vi "Rapid Target Adjustment.vi"(0 "Focus and Tracking":T4, 1 "Calibration":T2, 2 "Target":T1, 3 "System of Reference Interface":T3, 4 "Tip":T5, 5 "Error In":errorcluster, 6 "Step [um]":dbl=4.0, 7 "Contrast AVG frames number [unused]":i32=3, 10 "Max Distance [um]":dbl=100.0, 11 "Active":refnum<vi>, 12 "Start Coordinates [pix]":refnum<vi>, 13 "Abort":refnum<vi>) -> (14 "Fail":bool, 15 "Scope Error":bool, 17 "Aborted":bool, 18 "Optical Coordinates [um]":cluster{"X":dbl, "Y":dbl, "Z":dbl}, 19 "Error Out":errorcluster)   [LabVIEW 2012, in "Targeting Unit.lvlib"]
uses:
  Targeting Unit.lvlib
  <vilib>/Analysis/Matrix/Datatypes/RealMatrix.ctl
  <vilib>/Analysis/Matrix/NI_Matrix.lvlib
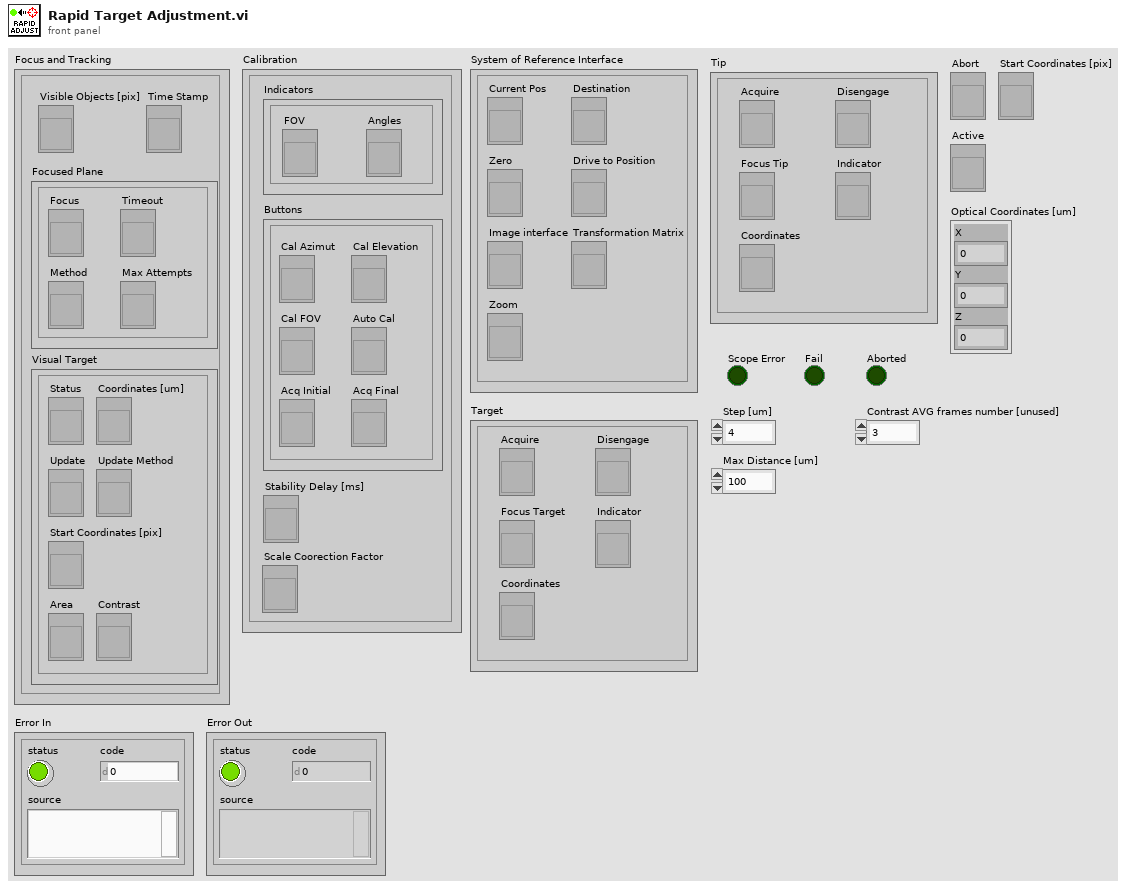
[diagram p1: front panel]
types:
  T1 = cluster{"Coordinates":refnum<vi>, "Acquire":refnum<vi>, "Disengage":refnum<vi>, "Indicator":refnum<vi>, "Focus Target":refnum<vi>}
  T2 = cluster{"Indicators":cluster{"FOV":refnum<vi>, "Angles":refnum<vi>}, "Buttons":cluster{"Cal FOV":refnum<vi>, "Cal Azimut":refnum<vi>, "Cal Elevation":refnum<vi>, "Auto Cal":refnum<vi>, "Acq Initial":refnum<vi>, "Acq Final":refnum<vi>}, "Stability Delay [ms]":refnum<vi>, "Scale Coorection Factor":refnum<vi>}
  T3 = cluster{"Current Pos":refnum<vi>, "Image interface":refnum<vi>, "Transformation Matrix":refnum<vi>, "Zero":refnum<vi>, "Destination":refnum<vi>, "Drive to Position":refnum<vi>, "Zoom":refnum<vi>}
  T4 = cluster{"Focused Plane":cluster{"Focus":refnum<vi>, "Timeout":refnum<vi>, "Max Attempts":refnum<vi>, "Method":refnum<vi>}, "Time Stamp":refnum<vi>, "Visual Target":cluster{"Coordinates [um]":refnum<vi>, "Status":refnum<vi>, "Update":refnum<vi>, "Update Method":refnum<vi>, "Start Coordinates [pix]":refnum<vi>, "Area":refnum<vi>, "Contrast":refnum<vi>}, "Visible Objects [pix]":refnum<vi>}
  T5 = cluster{"Coordinates":refnum<vi>, "Acquire":refnum<vi>, "Disengage":refnum<vi>, "Indicator":refnum<vi>, "Focus Tip":refnum<vi>}
  T6 = cluster{"X [um]":dbl, "Y [um]":dbl, "Z [um]":dbl}
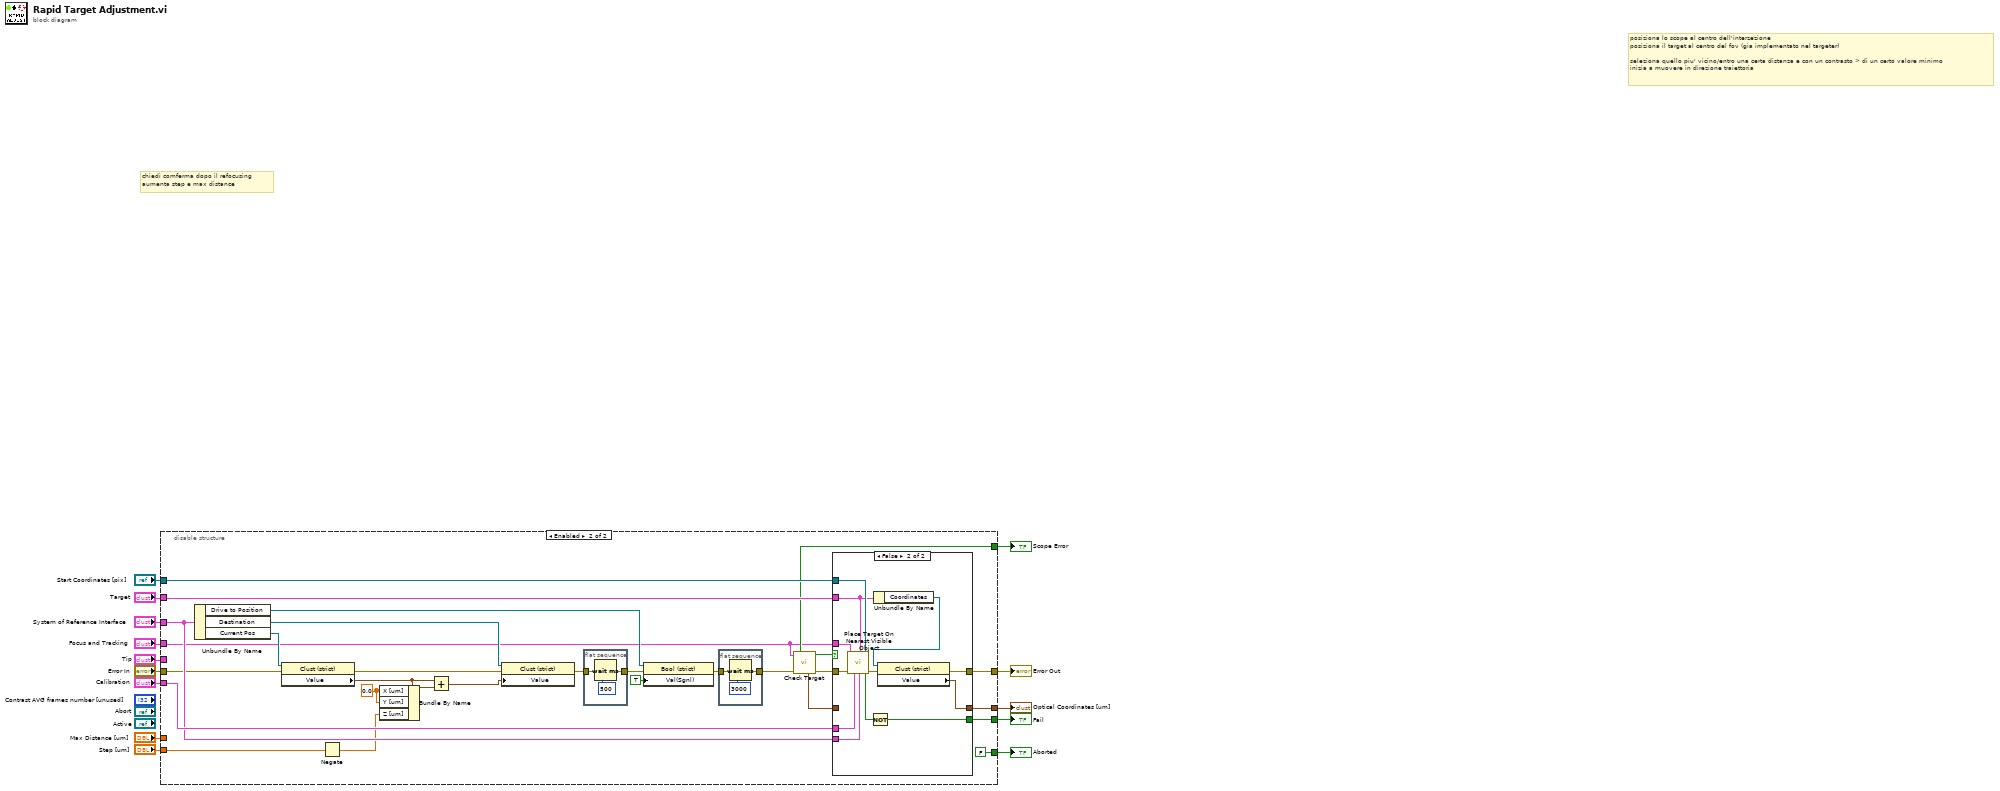
[diagram p0: block diagram]
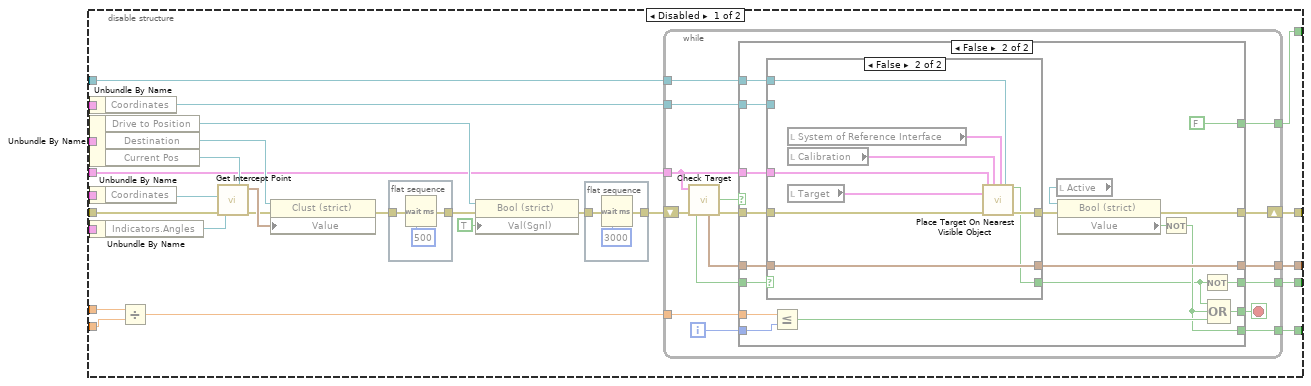
[diagram p2: hidden frame]
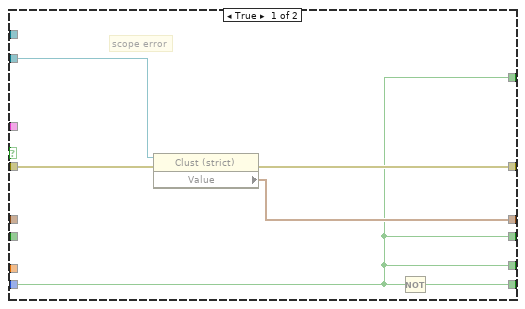
[diagram p3: hidden frame]
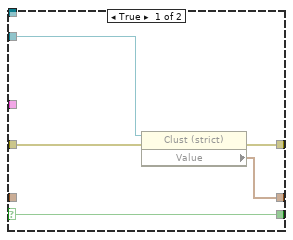
[diagram p4: hidden frame]
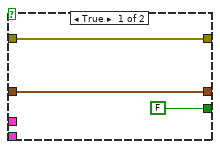
[diagram p5: hidden frame]
diagram:
  # "posiziona lo scope al centro dell'interzezione\nposiziona il target al centro del fov (gia implementato nel targeter)\n\nseleziona quello piu' vicino/entro una certa distanza e con un contrasto > di un certo valore minimo\ninizia a muovere in direzione traiettoria"
  # "chiedi comferma dopo il refocusing\naumenta step e max distance"
  n1 = disable-structure shown="Enabled" {
    disable-tunnel: "Step [um]" -> [w42 w112]
    disable-tunnel: "Max Distance [um]" -> [w41 _]
    disable-tunnel: "System of Reference Interface" -> [w40 w119]
    disable-tunnel: "Calibration" -> [w39 w120]
    disable-tunnel: "Tip" -> [w37 _]
    disable-tunnel: "Focus and Tracking" -> [w25 w102]
    disable-tunnel: [w24 FALSE ("Aborted")] -> w8
    disable-tunnel: [w23 w106] -> w7
    disable-tunnel: [w22 w127] -> w6
    disable-tunnel: "Target" -> [w21 w129]
    disable-tunnel: [w20 w105] -> w4
    disable-tunnel: [w19 w128] -> w3
    disable-tunnel: "Start Coordinates [pix]" -> [w15 w130]
    disable-tunnel: "Error In" -> [w26 w117]
    frame Disabled {
      n2 = Unbundle By Name(w21) -> ("Coordinates"=w18:refnum<vi>)
      n3 = Unbundle By Name(w40) -> ("Drive to Position"=w29:refnum<vi>, "Destination"=w30:refnum<vi>, "Current Pos"=w31:refnum<vi>)
      n4 = Unbundle By Name(w37) -> ("Coordinates"=w17:refnum<vi>)
      n5 = Unbundle By Name(w39) -> ("Indicators.Angles"=w27:refnum<vi>)
      n6 = Divide(x=w41, y=w42) -> (x/y=w38:dbl)
      n7 = call "Get Intercept Point.vi"("error in (no error)"=w26, "Current  System of Reference Position"=w31, "Tip Position"=w17, "Angles"=w27) -> ("error out"=w28:errorcluster, "Intercept Point"=w32:T6)  [unwired: 6 in]
      n8 = property class="Clust (strict)"(reference=w30, error in=w28, "Value"=w32) -> (error out=w35:errorcluster)  [unwired: 1 out]
      n9 = flat-sequence {
        tunnel: [w101] -> w34
        tunnel: w35 -> [w101]
        frame #0 {
          n10 = Wait (ms)(milliseconds to wait=u32 500) -> ()  [unwired: 1 out]
        }
      }
      n11 = property class="Bool (strict)"(reference=w29, error in=w34, "Val(Sgnl)"=TRUE ("Value")) -> (error out=w33:errorcluster)  [unwired: 1 out]
      n12 = flat-sequence {
        tunnel: [w99] -> w16
        tunnel: w33 -> [w99]
        frame #0 {
          n13 = Wait (ms)(milliseconds to wait=u32 3000) -> ()  [unwired: 1 out]
        }
      }
      n14 = while {
        shift-right: [w56] -> w19
        shift-left: w16 -> [w54]
        tunnel: w25 -> [w44]
        tunnel: w38 -> [w58]
        tunnel: [w46] -> w22
        tunnel: [w51] -> w24
        tunnel: [w49] -> w23
        tunnel: [w47] -> w20
        tunnel: w18 -> [w45]
        tunnel: w15 -> [w43]
        i -> [w57]
        stop <- w55 stop-if-true
        n15 = call "Check Target.vi"("Error In"=w54, "Focus and Tracking"=w44) -> ("Error out"=w53:errorcluster, "Scope Error"=w52:bool, "Target OK"=w50:bool, "Optical Coordinates [um]"=w48:cluster{"X":dbl, "Y":dbl, "Z":dbl})  [unwired: 3 in, 3 out]
        n16 = case shown="False" w52 {
          selector: w52 -> [w59 _]
          tunnel: w53 -> [w63 w78]
          tunnel: w58 -> [_ w83]
          tunnel: w57 -> [_ w82]
          tunnel: [w62 w81] -> w56
          tunnel: [w59 w80] -> w55
          tunnel: [w64 w69] -> w51
          tunnel: w50 -> [_ w71]
          tunnel: [w59 FALSE] -> w49
          tunnel: w48 -> [_ w72]
          tunnel: [w60 w73] -> w47
          tunnel: [w59 w74] -> w46
          tunnel: w45 -> [w61 w70]
          tunnel: w44 -> [_ w66]
          tunnel: w43 -> [_ w65]
          frame True {
            # "scope error"
            n17 = property class="Clust (strict)"(reference=w61, error in=w63) -> (error out=w62:errorcluster, "Value"=w60:T6)  [unwired: 1 out]
            n18 = Not(x=w59) -> (.not. x?=w64:bool)
          }
          frame False {
            n19 = case shown="False" w71 {
              selector: w71 -> [w88 _]
              tunnel: [w86 w96] -> w79
              tunnel: w78 -> [w87 w92]
              tunnel: [w85 w97] -> w73
              tunnel: w72 -> [_ w97]
              tunnel: [w88 w91] -> w68
              tunnel: w70 -> [w84 _]
              tunnel: w66 -> [_ w95]
              tunnel: w65 -> [_ w90]
              frame True {
                n20 = property class="Clust (strict)"(reference=w84, error in=w87) -> (error out=w86:errorcluster, "Value"=w85:T6)  [unwired: 1 out]
              }
              frame False {
                n21 = local read "System of Reference Interface"() -> (w93:T3)
                n22 = local read "Calibration"() -> (w94:T2)
                n23 = local read "Target"() -> (w89:T1)
                n24 = call "Place Target On Nearest Visible Object.vi"("Focus and Tracking"=w95, "Start Coordinates [pix]"=w90, "System of Reference Interface"=w93, "Calibration"=w94, "Target"=w89, "error in (no error)"=w92) -> ("Detected"=w91:bool, "error out"=w96:errorcluster)  [unwired: 8 in]
              }
            }
            n25 = Less Or Equal?(x=w83, y=w82) -> (x <= y?=w76:bool)
            n26 = local read "Active"() -> (w67:refnum<vi>)
            n27 = property class="Bool (strict)"(reference=w67, error in=w79) -> (error out=w81:errorcluster, "Value"=w77:bool)  [unwired: 1 out]
            n28 = Not(x=w77) -> (.not. x?=w69:bool)
            n29 = Not(x=w68) -> (.not. x?=w74:bool)
            n30 = Compound Arithmetic op=OR(w68, w69, w76) -> (w80:bool)
          }
        }
      }
    }
    frame Enabled {
      w111 = 0.0 ("X [um]")
      n31 = Unbundle By Name(w119) -> ("Drive to Position"=w121:refnum<vi>, "Destination"=w122:refnum<vi>, "Current Pos"=w118:refnum<vi>)
      n32 = property class="Clust (strict)"(reference=w118, error in=w117) -> (error out=w116:errorcluster, "Value"=w113:T6)  [unwired: 1 out]
      n33 = Negate(x=w112) -> (-x=w110:dbl)
      n34 = Bundle By Name(cluster=w113, "X [um]"=w111, "Y [um]"=w111, "Z [um]"=w110) -> (w114:T6)
      n35 = Add(x=w113, y=w114) -> (x+y=w115:T6)
      n36 = property class="Clust (strict)"(reference=w122, error in=w116, "Value"=w115) -> (error out=w125:errorcluster)  [unwired: 1 out]
      n37 = flat-sequence {
        tunnel: [w149] -> w124
        tunnel: w125 -> [w149]
        frame #0 {
          n38 = Wait (ms)(milliseconds to wait=u32 500) -> ()  [unwired: 1 out]
        }
      }
      n39 = property class="Bool (strict)"(reference=w121, error in=w124, "Val(Sgnl)"=TRUE ("Value")) -> (error out=w123:errorcluster)  [unwired: 1 out]
      n40 = flat-sequence {
        tunnel: [w147] -> w109
        tunnel: w123 -> [w147]
        frame #0 {
          n41 = Wait (ms)(milliseconds to wait=u32 3000) -> ()  [unwired: 1 out]
        }
      }
      n42 = call "Check Target.vi"("Error In"=w109, "Focus and Tracking"=w102) -> ("Error out"=w108:errorcluster, "Scope Error"=w106:bool, "Target OK"=w107:bool, "Optical Coordinates [um]"=w104:cluster{"X":dbl, "Y":dbl, "Z":dbl})  [unwired: 3 in, 3 out]
      n43 = case shown="False" w107 {
        tunnel: w130 -> [_ w145]
        tunnel: w102 -> [_ w144]
        tunnel: w129 -> [_ w137]
        tunnel: [w132 w135] -> w128
        tunnel: [FALSE w142] -> w127
        tunnel: w120 -> [_ w141]
        tunnel: w119 -> [_ w140]
        tunnel: w108 -> [w132 w139]
        tunnel: [w133 w134] -> w105
        tunnel: w104 -> [w133 _]
        frame True {
        }
        frame False {
          n44 = call "Place Target On Nearest Visible Object.vi"("Focus and Tracking"=w144, "Start Coordinates [pix]"=w145, "System of Reference Interface"=w140, "Calibration"=w141, "Target"=w137, "error in (no error)"=w139) -> ("Detected"=w143:bool, "error out"=w138:errorcluster)  [unwired: 8 in]
          n45 = Not(x=w143) -> (.not. x?=w142:bool)
          n46 = Unbundle By Name(w137) -> ("Coordinates"=w136:refnum<vi>)
          n47 = property class="Clust (strict)"(reference=w136, error in=w138) -> (error out=w135:errorcluster, "Value"=w134:T6)  [unwired: 1 out]
        }
      }
    }
  }
  "Error Out" <- w3
  "Scope Error" <- w7
  "Fail" <- w6
  "Aborted" <- w8
  "Optical Coordinates [um]" <- w4
